vi "Serial_readable.vi"(8 "error in (no error)":errorcluster, 11 "Serial in":refnum<class "Serial.lvclass">) -> (0 "error out":errorcluster, 2 "Readable":bool, 3 "Serial out":refnum<class "Serial.lvclass">)   [LabVIEW 2011, in "mbed_LVLibrary.lvlib" / "Serial.lvclass"]
doc: "Checks if there is data ready to be read from the mbed Serial port"
uses:
  Serial.lvclass
  Serial.lvclass/Serial.ctl
  Transport Mechanisms/mbed/mbed.lvclass
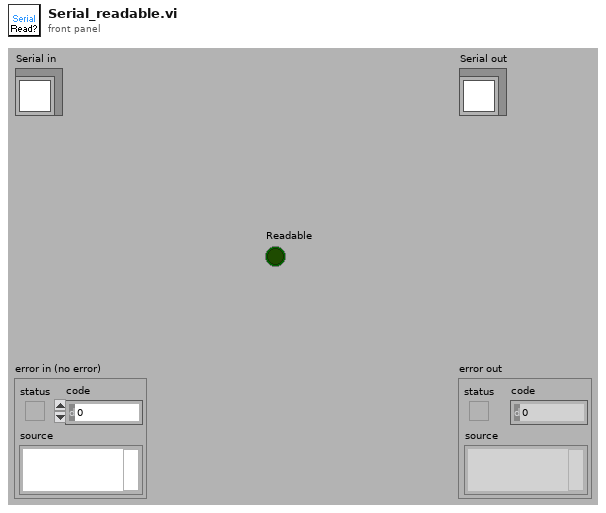
[diagram p1: front panel]
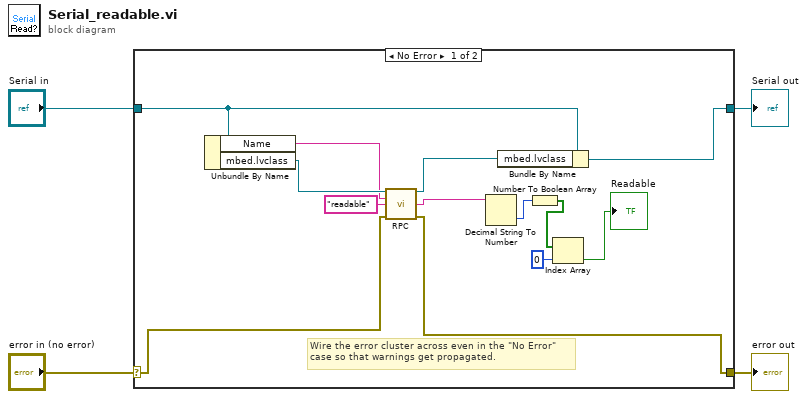
[diagram p0: block diagram]
diagram:
  n1 = case shown="No Error" "error in (no error)" {
    selector: "error in (no error)" -> [w6 w19]
    tunnel: [w5 w19] -> w3
    tunnel: [w8 w18] -> w1
    tunnel: "Serial in" -> [w9 w18]
    frame No Error {
      # "Wire the error cluster across even in the \"No Error\"\ncase so that warnings get propagated."
      n2 = Unbundle By Name(w9) -> ("Name"=w16:string, "mbed.lvclass"=w17:refnum<class "mbed.lvclass">)
      n3 = call-dynamic "RPC.vi"("mbed in"=w17, "Name"=w16, "method"="readable", "error in (no error)"=w6) -> ("mbed out"=w7:refnum<class "mbed.lvclass">, "RPC Result"=w14:string, "error out"=w5:errorcluster)  [unwired: 9 in]
      n4 = Decimal String To Number(string=w14) -> (number=w10:i32)  [unwired: 2 in, 1 out]
      n5 = Bundle By Name(cluster=w9, "mbed.lvclass"=w7) -> (w8:refnum<class "Serial.lvclass">)
      n6 = Number To Boolean Array(number=w10) -> (Boolean array=w12:bool[])
      n7 = Index Array(array=w12, index=0) -> (element=→"Readable":bool)
    }
    frame Error {
    }
  }
  "error out" <- w3
  "Serial out" <- w1
